vi "Get All Topics.vi"(8 "error in (no error)":errorcluster, 11 "TopicLookupTable":refnum<data-value>) -> (0 "error out":errorcluster, 2 "Topic Enqueuers":refnum<class "Message Enqueuer.lvclass">[](array[class]), 3 "TopicLookupTable":refnum<data-value>)   [LabVIEW 2017, in "Mediator.lvlib" / "TopicLookupTable.lvclass"]
doc: "<License>\nCopyright © 2017 Composed Systems, LLC | All rights reserved\nwww.composed.io\n\nAuthor: Ethan Stern <ethan.stern@composed.io>\n\nThis software is provided \"AS IS\" WITHOUT WARRANTIES, either express or implied, AND IS FOR EDUCATIONAL PURPOSES ONLY.\n</License>"
uses:
  TopicLookupTable.lvclass
  <vilib>/ActorFramework/Message Enqueuer/Message Enqueuer.lvclass
  TopicLookupTable.lvclass/TopicLookupTable.ctl
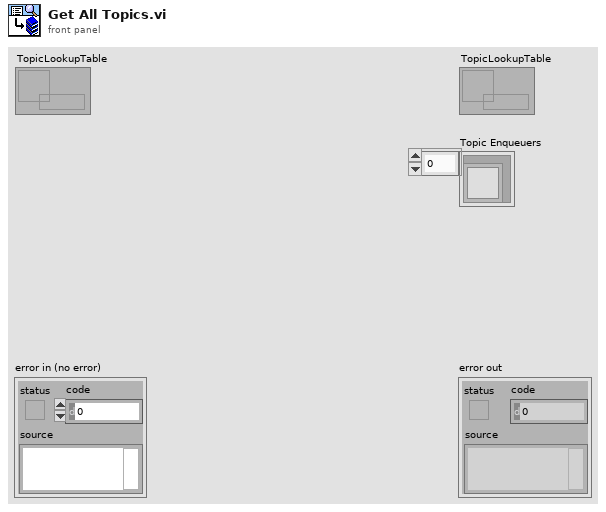
[diagram p1: front panel]
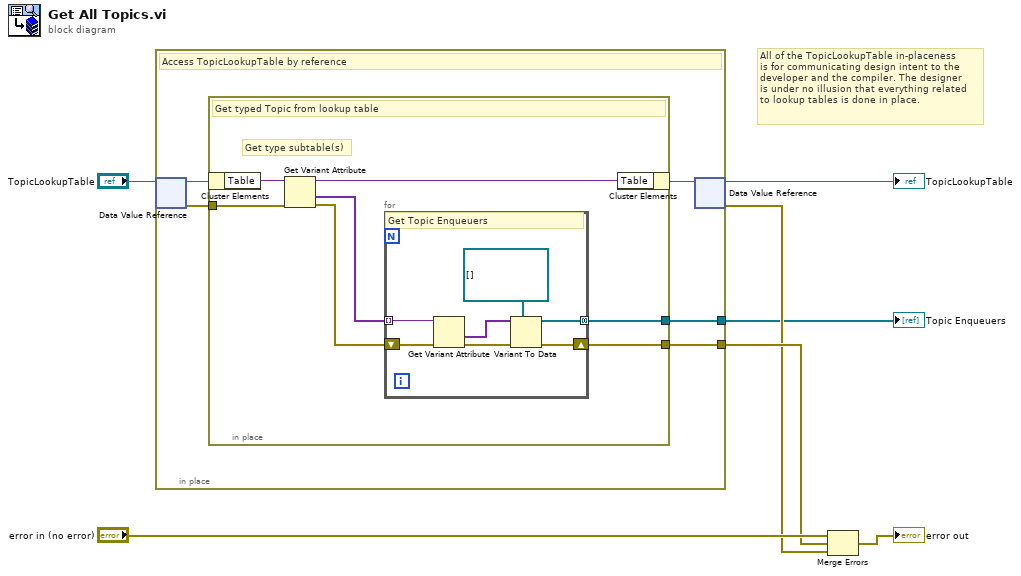
[diagram p0: block diagram]
diagram:
  # "All of the TopicLookupTable in-placeness\nis for communicating design intent to the\ndeveloper and the compiler. The designer\nis under no illusion that everything related\nto lookup tables is done in place."
  n1 = in-place {
    in-place-border: [w12] -> w4
    in-place-border: [w11] -> w1
    # "Access TopicLookupTable by reference"
    n2 = in-place-dvr #1("TopicLookupTable") -> (w10:refnum<class "TopicLookupTable.lvclass">, w8:errorcluster)
    n3 = in-place {
      in-place-border: [w14] -> w11
      in-place-border: [w13] -> w12
      in-place-border: w8 -> [w19]
      # "Get type subtable(s)"
      # "Get typed Topic from lookup table"
      n4 = in-place-cluster #2(w10) -> ("Table"=w18:variant)
      n5 = Get Variant Attribute(Variant=w18, error in=w19) -> (duplicate Variant=w16:variant, values=w17:variant[], error out=w15:errorcluster)  [unwired: 2 in, 1 out]
      n6 = for {
        tunnel: w17 -> [w26] mode=indexing
        shift-right: [w22] -> w13
        shift-left: w15 -> [w25]
        tunnel: [w20] -> w14 mode=concatenating
        # "Get Topic Enqueuers"
        n7 = Get Variant Attribute(Variant=w26, error in=w25) -> (values=w21:variant[], error out=w23:errorcluster)  [unwired: 2 in, 2 out]
        n8 = Variant To Data(error in=w23, type=refnum<class "Message Enqueuer.lvclass">[] [] ("Self Enqueuer"), Variant=w21) -> (data=w20:refnum<class "Message Enqueuer.lvclass">[], error out=w22:errorcluster)
      }
      n9 = in-place-cluster #2("Table"=w16) -> (w9:refnum<class "TopicLookupTable.lvclass">)
    }
    n10 = in-place-dvr #1(w9) -> (→"TopicLookupTable":refnum<data-value>, w3:errorcluster)
  }
  "Topic Enqueuers" <- w1
  n11 = Merge Errors("error in (no error)", w4, w3) -> (→"error out":errorcluster)
